vi "Find Open IP Port.vi"(8 "error in (no error)":errorcluster) -> (0 "error out":errorcluster, 3 "Port":u16)   [LabVIEW 2021, in "Networking_CIF_U.lvlib"]
uses:
  Networking_CIF_U.lvlib
  Typedef/Errors.ctl
  Errors/Append Error Location.vi
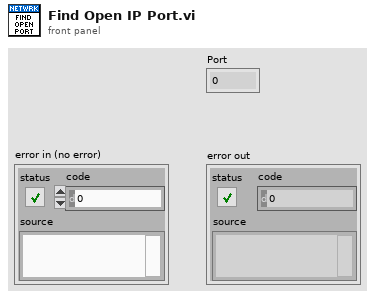
[diagram p1: front panel]
types:
  T1 = typedef "Networking_CIF_U.lvlib/Errors.ctl" = enum16{"Invalid IP Address", "No Subnet Match Found", "Error Finding Port", "No Ping Response", "Nettools Needed", "Error Checking Port"}
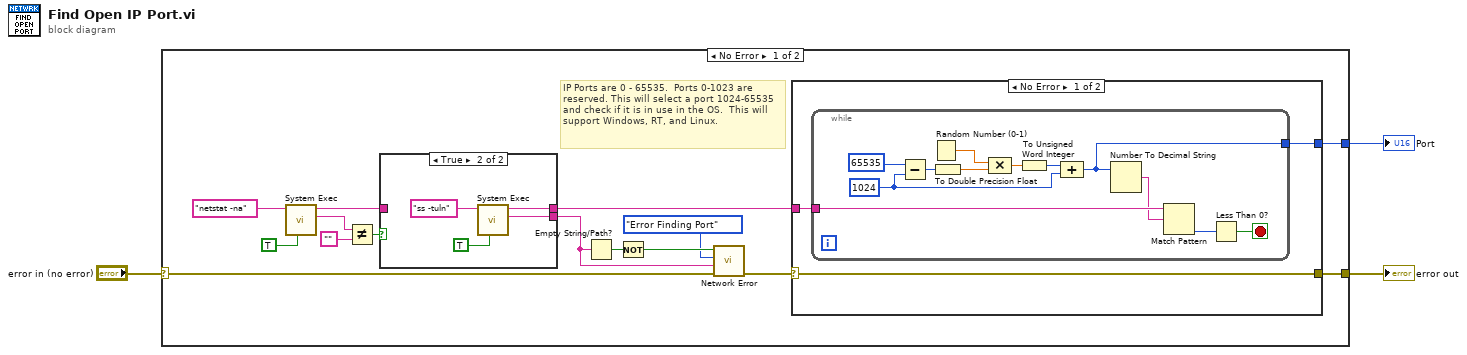
[diagram p0: block diagram]
diagram:
  n1 = case shown="No Error" "error in (no error)" {
    selector: "error in (no error)" -> [w17 w40]
    tunnel: [w4 w40] -> w3
    tunnel: [w18 _] -> w2
    frame No Error {
      # "IP Ports are 0 - 65535.  Ports 0-1023 are reserved. This will select a port 1024-65535 and check if it is in use in the OS.  This will support Windows, RT, and Linux."
      n2 = call <vilib>:"System Exec.vi"("run minimized? (F)"=TRUE, "command line"="netstat -na") -> ("standard error"=w11:string, "standard output"=w7:string)  [unwired: 6 in, 2 out]
      n3 = Not Equal?(x=w11, y="") -> (x != y?=w9:bool)
      n4 = case shown="True" w9 {
        tunnel: [_ w38] -> w15
        tunnel: w7 -> [w35 _]
        tunnel: [w35 w36] -> w6
        frame False {
        }
        frame True {
          n5 = call <vilib>:"System Exec.vi"("run minimized? (F)"=TRUE, "command line"="ss -tuln") -> ("standard error"=w38:string, "standard output"=w36:string)  [unwired: 6 in, 2 out]
        }
      }
      n6 = Empty String/Path?(string/path=w15) -> (empty?=w13:bool)
      n7 = Not(x=w13) -> (.not. x?=w16:bool)
      n8 = call "Network Error.vi"("error in (no error)"=w17, "String to Append"=w15, "Error"=Errors."Error Finding Port", "Insert Error"=w16) -> ("error out"=w5:errorcluster)  [unwired: 7 in]
      n9 = case shown="No Error" w5 {
        selector: w5 -> [w19 w34]
        tunnel: [w21 _] -> w18
        tunnel: w6 -> [w20 _]
        tunnel: [w19 w34] -> w4
        frame No Error {
          n10 = while {
            tunnel: [w22] -> w21
            tunnel: w20 -> [w26]
            stop <- w23 stop-if-true
            w27 = u16 1024
            n11 = Subtract(x=u16 65535, y=w27) -> (x-y=w32:u16)
            n12 = Random Number (0-1)() -> (number: 0 to 1=w30:dbl)
            n13 = To Double Precision Float(number=w32) -> (double precision float=w31:dbl)
            n14 = Compound Arithmetic op=MULTIPLY(w30, w31) -> (w29:dbl)
            n15 = To Unsigned Word Integer(number=w29) -> (unsigned 16bit integer=w28:u16)
            n16 = Compound Arithmetic op=ADD(w28, w27) -> (w22:u16)
            n17 = Number To Decimal String(number=w22) -> (decimal integer string=w25:string)  [unwired: 1 in]
            n18 = Match Pattern(string=w26, regular expression=w25) -> (offset past match=w24:i32)  [unwired: 1 in, 3 out]
            n19 = Less Than 0?(x=w24) -> (x < 0?=w23:bool)
          }
        }
        frame Error {
        }
      }
    }
    frame Error {
    }
  }
  "error out" <- w3
  "Port" <- w2
